vi "Connect.vi"(8 "error in (no error)":errorcluster, 11 "Bobcat 640 in":refnum<class "Bobcat 640.lvclass">) -> (0 "error out":errorcluster, 3 "Bobcat 640 out":refnum<class "Bobcat 640.lvclass">)   [LabVIEW 2018, in "Bobcat 640.lvlib" / "Bobcat 640.lvclass"]
uses:
  Bobcat 640.lvclass
  <vilib>/vision/driver/IMAQdx.llb/IMAQdx Camera Control Mode.ctl
  Bobcat 640.lvclass/Bobcat 640.ctl
  <vilib>/vision/driver/NI_Vision_Acquisition_Software.lvlib
  PPLs/Camera/Parent/Camera.lvlibp/Camera.lvclass
  C:/AME Test Engineering/LabVIEW/PPLs/Camera/Parent/Camera.lvlibp/Camera.lvclass
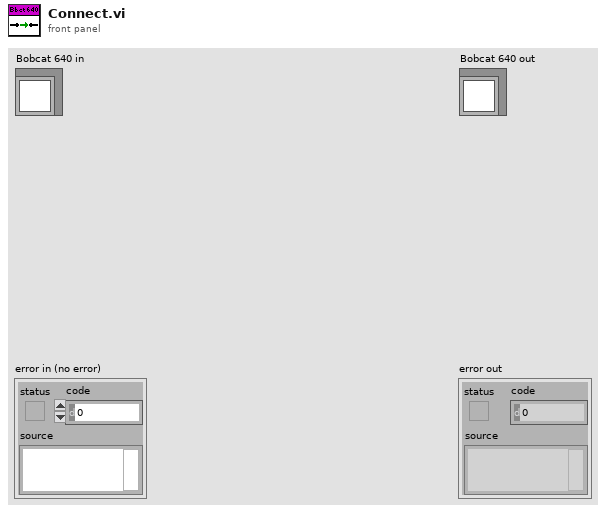
[diagram p1: front panel]
types:
  T1 = typedef "NI_Vision_Acquisition_Software.lvlib/IMAQdx Camera Control Mode.ctl" = enum32{"Controller", "Listener"}
  T2 = typedef "IMAQ Image.ctl" = refnum<image>
  T3 = typedef "Image Type" = u32
  T4 = typedef "IMAQdx.ctl" = refnum<k21>
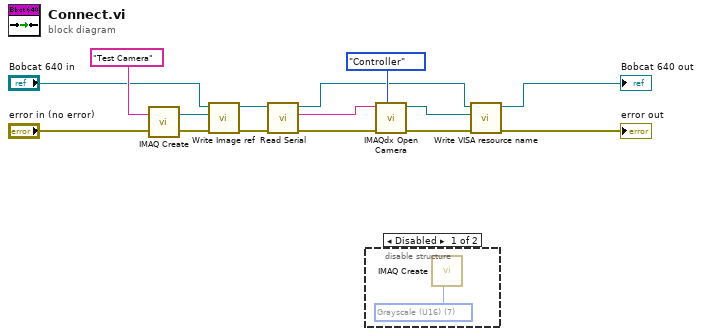
[diagram p0: block diagram]
diagram:
  n1 = call "IMAQ Create"("Image Name"="Test Camera", "error in (no error)"="error in (no error)") -> ("New Image"=w4:T2, "error out"=w6:errorcluster)  [unwired: 3 in]
  n2 = call "Write Image ref.vi"("error in (no error)"=w6, "Image"=w4, "Camera in"="Bobcat 640 in") -> ("error out"=w2:errorcluster, "Camera out"=w1:refnum<class "Bobcat 640.lvclass">)  [unwired: 7 in]
  n3 = call "Read Serial.vi"("error in (no error)"=w2, "Camera in"=w1) -> ("error out"=w8:errorcluster, "Serial"=w10:string, "Camera out"=w9:refnum<class "Bobcat 640.lvclass">)  [unwired: 7 in]
  n4 = disable-structure shown="Disabled" {
    frame Disabled {
      w16 = T3 7 items=["Grayscale (U8)", "Grayscale (I16)", "Grayscale (SGL)", "Complex (CSG)", "RGB (U32)", "HSL (U32)", "RGB (U64)", "Grayscale (U16)"] ("Image Type")
      n5 = call "IMAQ Create"("Image Type"=w16) -> ()  [unwired: 4 in, 2 out]
    }
    frame Enabled {
    }
  }
  n6 = call <vilib>:"IMAQdx Open Camera.vi"("Camera Control Mode"=IMAQdx_Camera_Control_Mode."Controller", "error in"=w8, "Session In"=w10) -> ("error out"=w15:errorcluster, "Session Out"=w13:T4)  [unwired: 7 in]
  n7 = call "Write VISA resource name.vi"("error in (no error)"=w15, "IMAQdx Session"=w13, "Bobcat 640 in"=w9) -> ("error out"=→"error out":errorcluster, "Bobcat 640 out"=→"Bobcat 640 out":refnum<class "Bobcat 640.lvclass">)  [unwired: 7 in]
